vi "NXT_MIDBRAIN_BEHAVIOR Master Brain.vi"(4 "_sensorData":T2={"_irData"={"_irDistance"=0, "_irHeading"=0, "_irTimestamp"=0}, "_batteryVoltage"=0, "_NXTButtonStates"=[FALSE, FALSE, FALSE]}, 5 "_fromPC":u8[](array[numeric])=[0, 0, 0, 0, 0, 0, 0, 0, 0, 0, 0], 6 "Previous Motor Position":T1={"_rudderCommand"=7, "_propCommand"=7, "_irServoCommand"=7}, 7 "_behaviorWeights":T5=[0, 0, 0, 0, 0, 0]) -> (0 "_irTheta":i8, 1 "_behaviorData":T4[](array[typedef]))   [LabVIEW 2012, in "Tugboat.lvrbt"]
uses:
  Tugboat.lvrbt
  behaviorWeights_t.ctl
  behaviorOutput_t.ctl
  motorCommands_t.ctl
  sensorData_t.ctl
  irData_t.ctl
panel:
  in  "_motorCommands":T1={"_rudderCommand"=7, "_propCommand"=7, "_irServoCommand"=7}
  # "L\nE\nF\nT"
  # "C\nE\nN\nT\nE\nR"
  # "R\nI\nG\nH\nT"
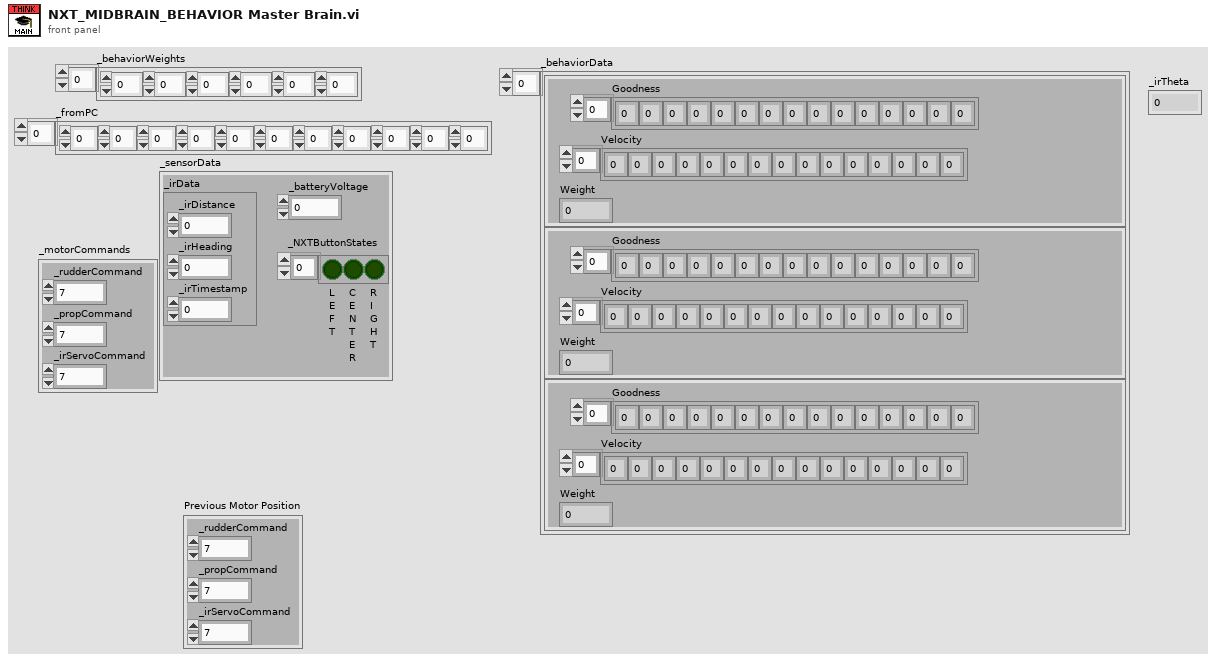
[diagram p1: front panel]
types:
  T1 = typedef "motorCommands_t.ctl" = cluster{"_rudderCommand":i8, "_propCommand":i8, "_irServoCommand":i8}
  T2 = typedef "sensorData_t.ctl" = cluster{"_irData":T3, "_batteryVoltage":i32, "_NXTButtonStates":bool[]}
  T3 = typedef "irData_t.ctl" = cluster{"_irDistance":i32, "_irHeading":i32, "_irTimestamp":u32}
  T4 = typedef "behaviorOutput_t.ctl" = cluster{"Goodness":i8[], "Velocity":i8[], "Weight":i8}
  T5 = typedef "behaviorWeights_t.ctl" = i8[]
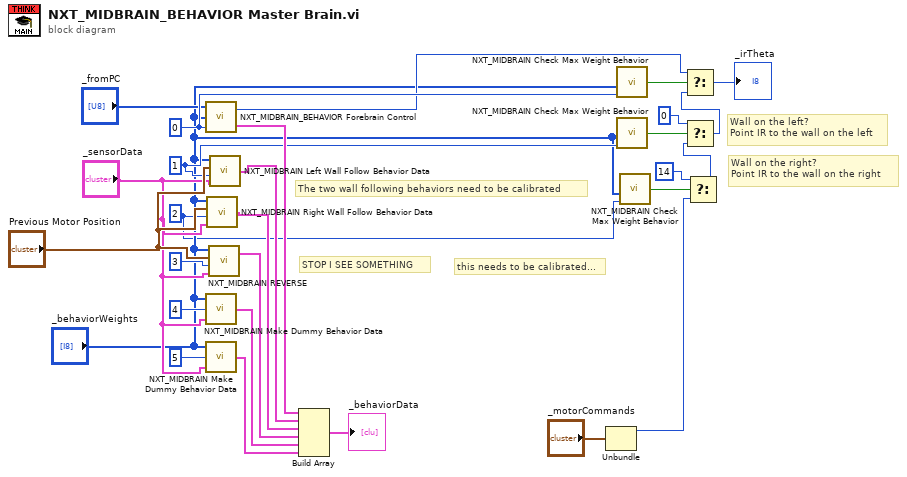
[diagram p0: block diagram]
diagram:
  w1 = 2 ("Behavior #")
  w21 = 0 ("Behavior #")
  w8 = 1 ("Behavior #")
  # "The two wall following behaviors need to be calibrated"
  # "this needs to be calibrated..."
  # "Wall on the right? \nPoint IR to the wall on the right"
  # "Wall on the left? \nPoint IR to the wall on the left"
  # "STOP I SEE SOMETHING"
  n1 = call "NXT_MIDBRAIN_BEHAVIOR Forebrain Control.vi"("Behavior #"=w21, "_behaviorWeights"="_behaviorWeights", "_fromPC"="_fromPC") -> ("_behaviorOutput"=w26:T4, "_FBirTheta"=w17:i8)
  n2 = call "NXT_MIDBRAIN Make Dummy Behavior Data.vi"("_sensorData"="_sensorData", "Behavior #"=4, "Behavior Weights"="_behaviorWeights") -> ("Behavior Output"=w25:T4)
  n3 = call "NXT_MIDBRAIN Make Dummy Behavior Data.vi"("_sensorData"="_sensorData", "Behavior #"=5, "Behavior Weights"="_behaviorWeights") -> ("Behavior Output"=w24:T4)
  n4 = call "NXT_MIDBRAIN Right Wall Follow Behavior Data.vi"("_sensorData"="_sensorData", "Behavior #"=w1, "Previous Motor Position"="Previous Motor Position", "Behavior Weights"="_behaviorWeights") -> ("Behavior Output"=w11:T4)
  n5 = call "NXT_MIDBRAIN REVERSE.vi"("_sensorData"="_sensorData", "Behavior #"=3, "Previous Motor Position"="Previous Motor Position", "Behavior Weights"="_behaviorWeights") -> ("Behavior Output"=w13:T4)  [unwired: 1 out]
  n6 = call "NXT_MIDBRAIN Left Wall Follow Behavior Data.vi"("_sensorData"="_sensorData", "Behavior #"=w8, "Previous Motor Position"="Previous Motor Position", "Behavior Weights"="_behaviorWeights") -> ("Behavior Output"=w10:T4)
  n7 = Build Array(w26, w10, w11, w13, w25, w24) -> (→"_behaviorData":T4[])
  n8 = Unbundle("_motorCommands") -> ("_rudderCommand"=w3:i8)  [unwired: 2 out]
  n9 = call "NXT_MIDBRAIN Check Max Weight Behavior.vi"("Behavior #"=w21, "_behaviorWeights"="_behaviorWeights") -> ("Max?"=w18:bool)  [unwired: 2 in]
  n10 = call "NXT_MIDBRAIN Check Max Weight Behavior.vi"("Behavior #"=w8, "_behaviorWeights"="_behaviorWeights") -> ("Max?"=w22:bool)  [unwired: 2 in]
  n11 = call "NXT_MIDBRAIN Check Max Weight Behavior.vi"("Behavior #"=w1, "_behaviorWeights"="_behaviorWeights") -> ("Max?"=w6:bool)  [unwired: 2 in]
  n12 = Select(t=i8 14, s=w6, f=w3) -> (s? t:f=w4:i8)
  n13 = Select(t=i8 0, s=w22, f=w4) -> (s? t:f=w15:i8)
  n14 = Select(t=w17, s=w18, f=w15) -> (s? t:f=→"_irTheta":i8)
